vi "Send ConnectionInfoUpdated.vi"(7 "Message Priority (Normal)":T2=enum."Normal", 8 "error in (no error)":errorcluster, 10 "Connection Information":T1={"Connection number"=-1, "Remote Address"="", "Remote Port"=0, "Connection ID"=refnum, "bytes received"=0, "bytes  sent"=0}, 11 "Message Enqueuer":refnum<class "Message Enqueuer.lvclass">) -> (0 "error out":errorcluster, 3 "Message Enqueuer out":refnum<class "Message Enqueuer.lvclass">)   [LabVIEW 2023, in "TCP_Server_Connection_Handler.lvlib" / "ConnectionInfoUpdated Msg.lvclass"]
doc: "This VI sends the message to an actor."
uses:
  ConnectionInfoUpdated Msg.lvclass
  ConnectionInfoUpdated Msg.lvclass/ConnectionInfoUpdated Msg.ctl
  <vilib>/ActorFramework/Message Enqueuer/Message Enqueuer.lvclass
  C:/Program Files (x86)/National Instruments/LabVIEW 2023/vi.lib/ActorFramework/Message/Message.lvclass
  C:/Source/LabVIEW/TCP_server/TCP_Server_Connection_Handler/TCP_Connections_Controller Messages/ConnectionInfoUpdated Msg/ConnectionInfoUpdated Msg.lvclass
  <vilib>/ActorFramework/Message Enqueuer/Message Priority.ctl
  TCP_Listener/TypeDefinitions/ConnectionInformation.ctl
  TCP_Listener/TCP_Listener.lvlib
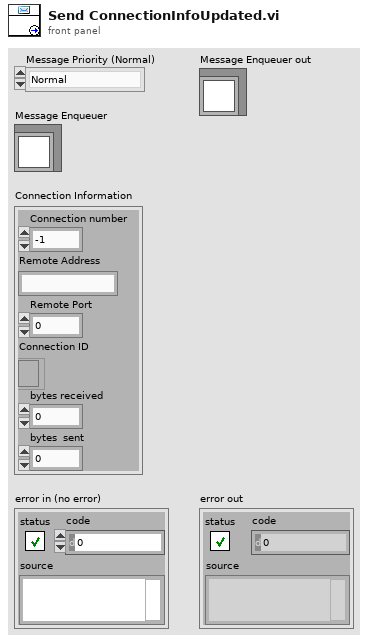
[diagram p1: front panel]
types:
  T1 = typedef "TCP_Listener.lvlib/ConnectionInformation.ctl" = cluster{"Connection number":i32, "Remote Address":string, "Remote Port":u16, "Connection ID":refnum<k5>, "bytes received":i32, "bytes  sent":i32}
  T2 = typedef "Actor Framework.lvlib/Message Enqueuer.lvclass/Message Priority.ctl" = enum16{"Low", "Normal", "High"}
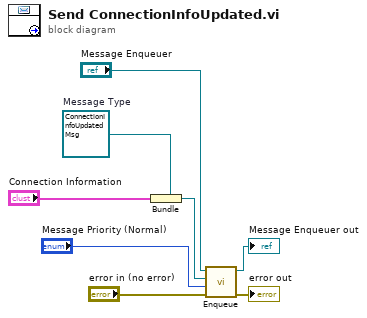
[diagram p0: block diagram]
diagram:
  w5 = refnum<class "ConnectionInfoUpdated Msg.lvclass"> refnum  # Message Type
  n1 = Bundle(cluster=w5, "Connection Information") -> (w4:refnum<class "ConnectionInfoUpdated Msg.lvclass">)
  n2 = call <vilib>:"Enqueue.vi"("error in (no error)"="error in (no error)", "Message Priority (Normal)"="Message Priority (Normal)", "Message"=w4, "Message Enqueuer in"="Message Enqueuer") -> ("error out"=→"error out":errorcluster, "Message Enqueuer in"=→"Message Enqueuer out":refnum<class "Message Enqueuer.lvclass">)  [unwired: 6 in]
